vi "_UnitTest.ClusterToArray.vi"() -> ()   [LabVIEW 2017]
panel:
  out "Cluster 2":variant
  out "Array 2":variant[](array[variant])
  out "Cluster":variant
  out "Array":variant[](array[variant])
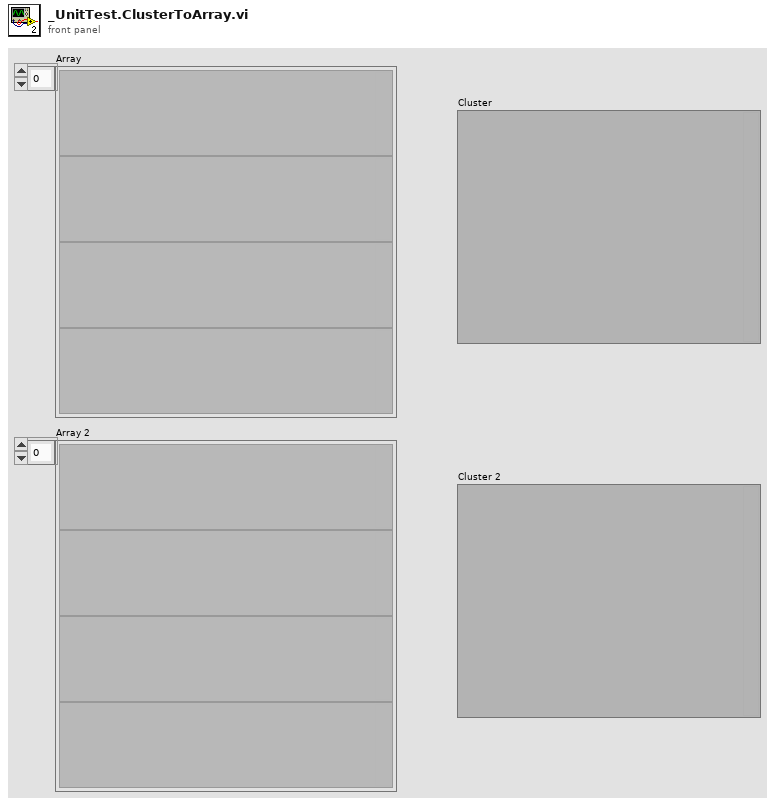
[diagram p1: front panel]
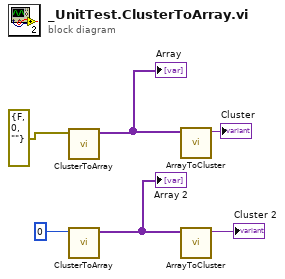
[diagram p0: block diagram]
diagram:
  n1 = call "ClusterToArray.vi"("Cluster"=errorcluster {"status"=FALSE, "code"=0, "source"=""} ("error in (no error)")) -> ("Array"=w5:variant[])  [unwired: 10 in]
  "Array" <- w5
  n2 = call "ClusterToArray.vi"("Cluster"=0 ("code")) -> ("Array"=w2:variant[])  [unwired: 10 in]
  "Array 2" <- w2
  n3 = call "ArrayToCluster.vi"("Array"=w5) -> ("Cluster"=→"Cluster":variant)  [unwired: 10 in]
  n4 = call "ArrayToCluster.vi"("Array"=w2) -> ("Cluster"=→"Cluster 2":variant)  [unwired: 10 in]
